vi "Get Acquired Data.vi"(8 "error in (no error)":errorcluster, 11 "CCDCamera in":refnum<class "Simulated_CCD_Camera.lvclass">) -> (0 "error out":errorcluster, 3 "CCDCamera out":refnum<class "Simulated_CCD_Camera.lvclass">)   [LabVIEW 2018, in "Simulated_CCD_Camera.lvclass"]
uses:
  Simulated_CCD_Camera.lvclass
  Simulated_CCD_Camera.lvclass/Simulated_CCD_Camera.ctl
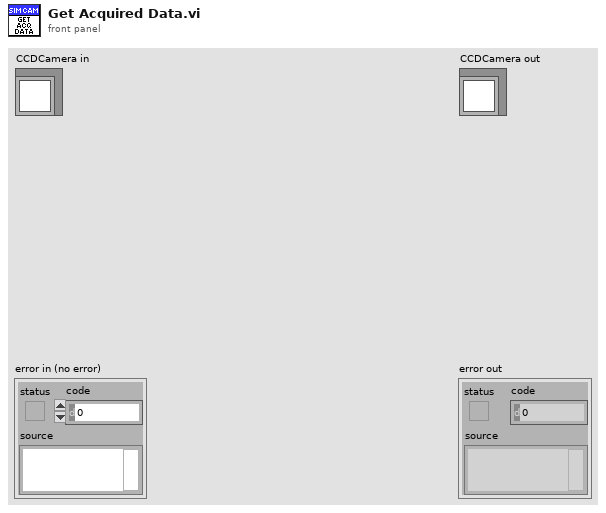
[diagram p1: front panel]
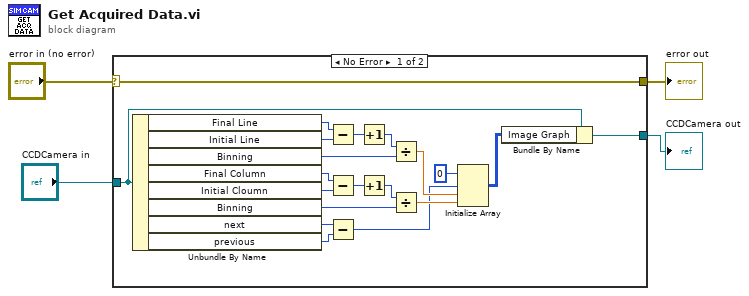
[diagram p0: block diagram]
diagram:
  n1 = case shown="No Error" "error in (no error)" {
    selector: "error in (no error)" -> [w12 w26]
    tunnel: [w12 w26] -> w1
    tunnel: [w24 w25] -> w2
    tunnel: "CCDCamera in" -> [w6 w25]
    frame No Error {
      n2 = Unbundle By Name(w6) -> ("Final Line"=w23:u16, "Initial Line"=w22:u16, "Binning"=w16:u16, "Final Column"=w21:u16, "Initial Cloumn"=w20:u16, "Binning"=w14:u16, "next"=w5:u16, "previous"=w7:u16)
      n3 = Subtract(x=w23, y=w22) -> (x-y=w19:u16)
      n4 = Subtract(x=w21, y=w20) -> (x-y=w18:u16)
      n5 = Subtract(x=w5, y=w7) -> (x-y=w8:u16)
      n6 = Increment(x=w19) -> (x+1=w17:u16)
      n7 = Increment(x=w18) -> (x+1=w15:u16)
      n8 = Divide(x=w17, y=w16) -> (x/y=w11:dbl)
      n9 = Divide(x=w15, y=w14) -> (x/y=w10:dbl)
      n10 = Initialize Array(u16 0, w8, w11, w10) -> (w9:u16[][][])
      n11 = Bundle By Name(cluster=w6, "Image Graph"=w9) -> (w24:refnum<class "Simulated_CCD_Camera.lvclass">)
    }
    frame Error {
    }
  }
  "error out" <- w1
  "CCDCamera out" <- w2
